vi "MeasurementServer_GetRequest_Register.vi"(0 "gRPCid":T1, 3 "error in (no error)":errorcluster) -> (7 "gRPCid out":T1, 9 "eventname":string, 10 "error out":errorcluster)   [LabVIEW 2019, in "labview-grpc-measurement-server.lvlib"]
uses:
  labview-grpc-measurement-server.lvlib
  MeasurementServer_gRPCid.ctl
  MeasurementServer_RegisterRequest.ctl
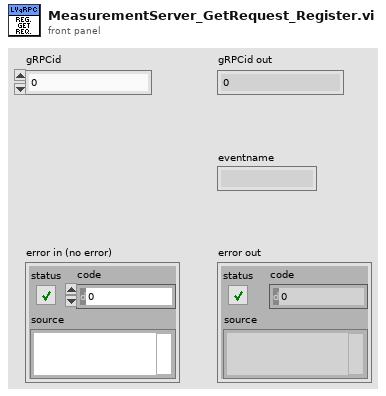
[diagram p1: front panel]
types:
  T1 = typedef "labview-grpc-measurement-server.lvlib/MeasurementServer_gRPCid.ctl" = u64
  T2 = typedef "labview-grpc-measurement-server.lvlib/MeasurementServer_RegisterRequest.ctl" = cluster{"eventname":string}
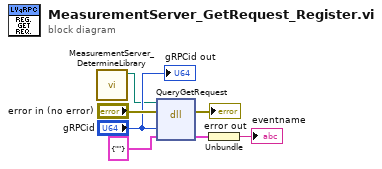
[diagram p0: block diagram]
diagram:
  n1 = call "MeasurementServer_DetermineLibrary.vi"() -> ("path out"=w1:path)  [unwired: 11 in]
  n2 = dll-call lib="C:/Users/chericks/Desktop/LabVIEW-grpc-measurement-server/build/Debug/labview_measurement_server.dll" fn="QueryGetRequest"(path in=w1, error in="error in (no error)", "id"="gRPCid", "data"=T2 {"eventname"=""} ("RegistrationRequest")) -> (error out=→"error out":errorcluster, "data"=w3:T2)  [unwired: 3 in, 1 out]
  n3 = Unbundle(w3) -> ("eventname"=→"eventname":string)
  "gRPCid out" <- "gRPCid"
